vi "Mouse Move.vi"(8 "error in (no error)":errorcluster, 10 "Cell Position":T1, 11 "MCLB_Template in":refnum<class "MCLB_Template.lvclass">) -> (0 "error out":errorcluster, 3 "MCLB_Template out":refnum<class "MCLB_Template.lvclass">)   [LabVIEW 2021, in "MCLB_Template.lvclass"]
uses:
  MCLB_Template.lvclass
  MCLB_Template.lvclass/MCLB_Template.ctl
  <userlib>/_OpenG.lib/array/array.llb/Remove Duplicates from 1D Array (I32)__ogtk.vi
  <vilib>/Utility/miscctls.llb/LVRowAndColumnTypeDef.ctl
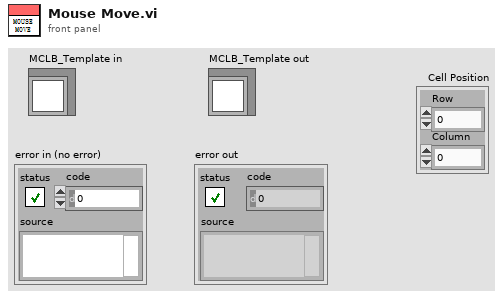
[diagram p1: front panel]
types:
  T1 = typedef "LVRowAndColumnTypeDef.ctl" = cluster{"Row":i32, "Column":i32}
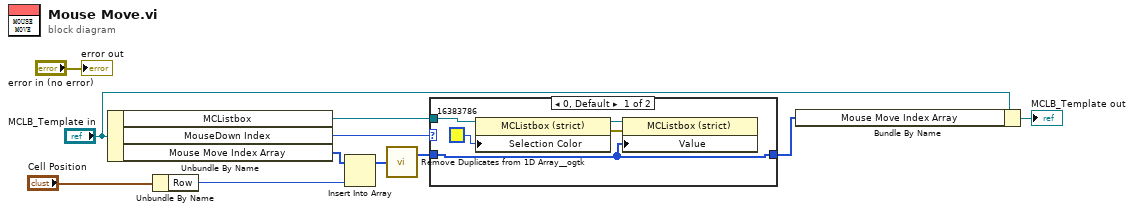
[diagram p0: block diagram]
diagram:
  n1 = Unbundle By Name("MCLB_Template in") -> ("MCListbox"=w4:refnum<vi>, "MouseDown Index"=w5:i32, "Mouse Move Index Array"=w8:i32[])
  n2 = Unbundle By Name("Cell Position") -> ("Row"=w7:i32)
  n3 = Insert Into Array(array=w8, new element=w7) -> (w9:i32[])  [unwired: 1 in]
  n4 = call-poly <userlib>:"Remove Duplicates from 1D Array__ogtk.vi"("Input Array"=w9) -> ("Output Array"=w3:i32[])  [unwired: 1 out]
  n5 = case shown="0, Default" w5 {
    tunnel: w4 -> [w13 _]
    tunnel: w3 -> [w12 w17]
    tunnel: [w12 w17] -> w1
    frame 0, Default {
      n6 = property on="Property Node" class="MCListbox (strict)"(reference=w13, "Selection Color"=u32 16383786) -> (reference out=w15:refnum<vi>, error out=w16:errorcluster)  [unwired: 1 in]
      n7 = property on="Property Node" class="MCListbox (strict)"(reference=w15, error in=w16, "Value"=w12) -> ()  [unwired: 2 out]
    }
    frame -1 {
    }
  }
  n8 = Bundle By Name(cluster="MCLB_Template in", "Mouse Move Index Array"=w1) -> (→"MCLB_Template out":refnum<class "MCLB_Template.lvclass">)
  "error out" <- "error in (no error)"
